vi "USR_TIME_FRU_REF_2 Read.vi"(4 "error in (no error)":errorcluster, 6 "Container State":T2, 7 "Display State In":T1) -> (0 "error out":errorcluster, 2 "Value":refnum<vi>, 3 "Display State Out":T1)   [LabVIEW 2014, in "Xgraph.xctl"]
uses:
  Xgraph.xctl
  <vilib>/_xctls/Container State.ctl
  State.ctl
  <vilib>/_xctls/XControlSupport.lvlib
panel:
  # "Replace the Value Indicator below with an Indicator of desired type.\nDo not remove this Indicator or the others from the connector pane. \nDo not change the connector pane pattern.\nThe Value Indicator should always be the second terminal from top on the output side in the connector pane."
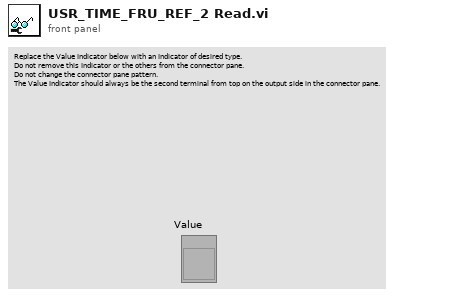
[diagram p1: front panel]
types:
  T1 = typedef "Xgraph.xctl/State.ctl" = cluster{"ʱƵ1":refnum<vi>, "ʱƵ2":refnum<vi>, "Cho1":refnum<vi>, "Cho2":refnum<vi>}
  T2 = typedef "XControlSupport.lvlib/Container State.ctl" = cluster{"Indicator?":bool, "Run Mode?":bool, " Refnum":refnum<vi>}
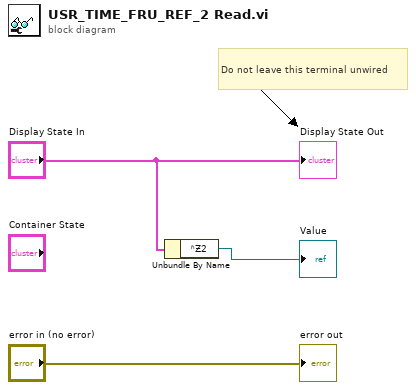
[diagram p0: block diagram]
diagram:
  # "Do not leave this terminal unwired"
  n1 = Unbundle By Name("Display State In") -> ("ʱƵ2"=→"Value":refnum<vi>)
  "error out" <- "error in (no error)"
  "Display State Out" <- "Display State In"
